vi "StoreChannelNameParams.vi"(4 "iNameBufferSize":i32, 6 "iIndex":i32, 8 "error in (no error)":errorcluster, 11 "ClassIn":refnum<class "NISTFGenPluginsBase.lvclass">) -> (0 "error out":errorcluster, 3 "ClassOut":refnum<class "NISTFGenPluginsBase.lvclass">)   [LabVIEW 2014, in "FGenPlugins.lvlib" / "NISTFGenPluginsBase.lvclass"]
uses:
  NISTFGenPluginsBase.lvclass
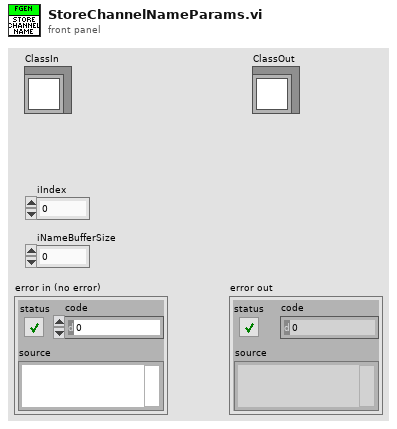
[diagram p1: front panel]
types:
  T1 = typedef "FGenPlugins.lvlib/NISTFGenPluginsBase.lvclass/ChannelParamElement.ctl" = cluster{"sName":string, "eOperateMode":u16, "bEnabled":bool, "eOutputMode":u16, "iIndex":i32, "iNameBufferSize":i32, "fGain":dbl}
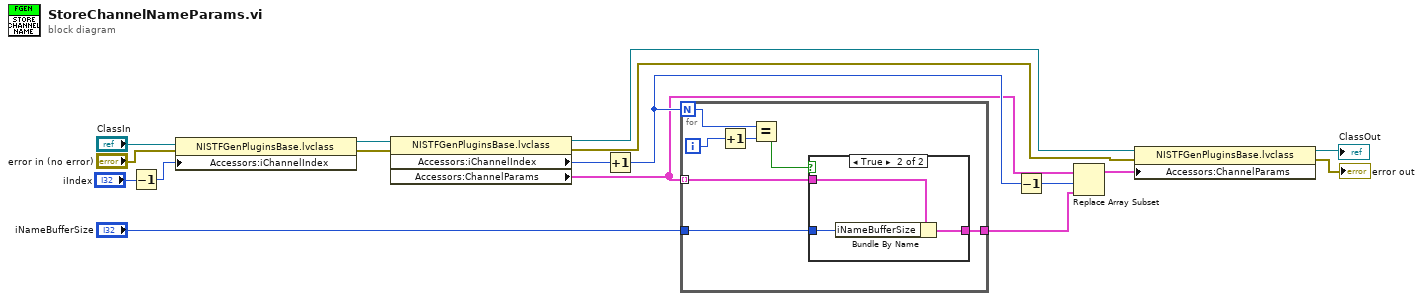
[diagram p0: block diagram]
diagram:
  n1 = Decrement(x="iIndex") -> (x-1=w1:i32)
  n2 = property class="NISTFGenPluginsBase.lvclass"(reference="ClassIn", error in="error in (no error)", "Accessors:iChannelIndex"=w1) -> (reference out=w5:refnum<class "NISTFGenPluginsBase.lvclass">, error out=w4:errorcluster)
  n3 = property class="NISTFGenPluginsBase.lvclass"(reference=w5, error in=w4) -> (reference out=w9:refnum<class "NISTFGenPluginsBase.lvclass">, error out=w8:errorcluster, "Accessors:iChannelIndex"=w12:i32, "Accessors:ChannelParams"=w7:T1[])
  n4 = Increment(x=w12) -> (x+1=w11:i32)
  n5 = for {
    N: w11 -> [w24]
    tunnel: w7 -> [w22] mode=indexing
    tunnel: [w21] -> w17
    tunnel: "iNameBufferSize" -> [w20]
    i -> [w19]
    n6 = Increment(x=w19) -> (x+1=w18:i32)
    n7 = Equal?(x=w24, y=w18) -> (x = y?=w23:bool)
    n8 = case shown="True" w23 {
      tunnel: w22 -> [w25 w28]
      tunnel: [w25 w27] -> w21
      tunnel: w20 -> [_ w26]
      frame False {
      }
      frame True {
        n9 = Bundle By Name(cluster=w28, "iNameBufferSize"=w26) -> (w27:T1)
      }
    }
  }
  n10 = Decrement(x=w11) -> (x-1=w10:i32)
  n11 = Replace Array Subset(array=w7, new element=w17, index=w10) -> (w16:T1[])
  n12 = property class="NISTFGenPluginsBase.lvclass"(reference=w9, error in=w8, "Accessors:ChannelParams"=w16) -> (reference out=→"ClassOut":refnum<class "NISTFGenPluginsBase.lvclass">, error out=→"error out":errorcluster)
